vi "extract full and sub movement sequences.vi"(8 "end points in":i32[](array[numeric]), 9 "Start points in":i32[](array[numeric]), 11 "player movement data":i32[](array[numeric])) -> (2 "Sub patterns":string[](array[string]), 3 "Full movement patterns":string[](array[string]))   [LabVIEW 2013]
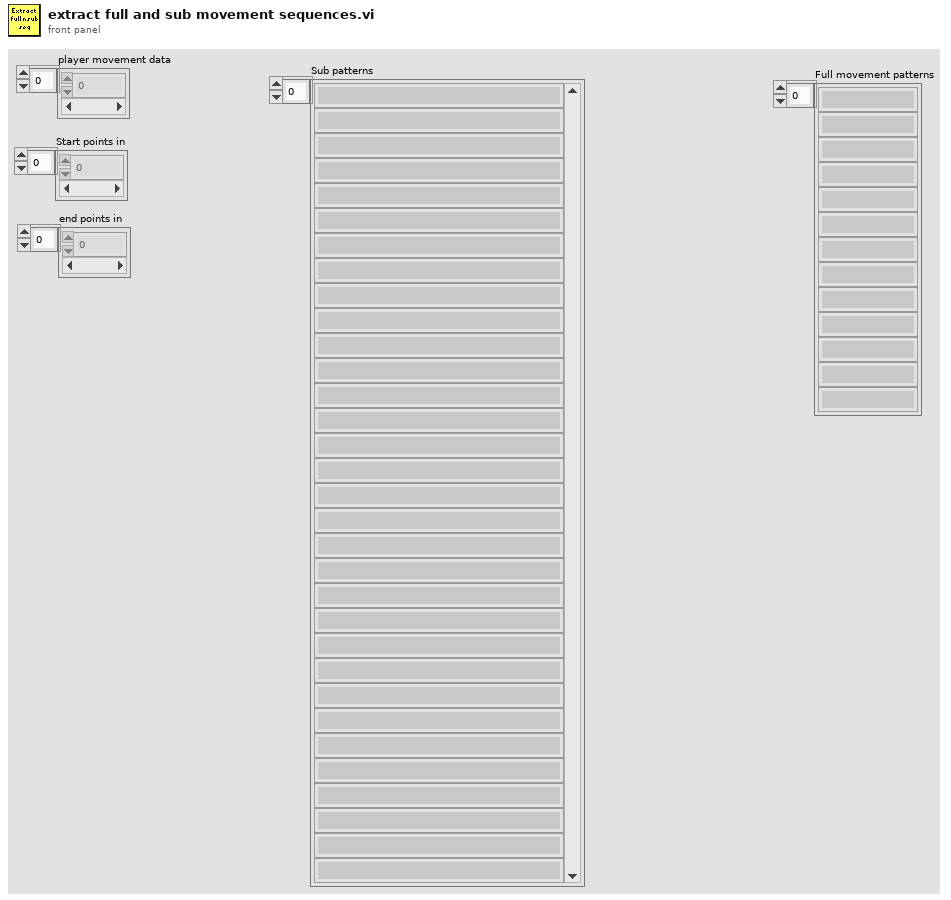
[diagram p1: front panel]
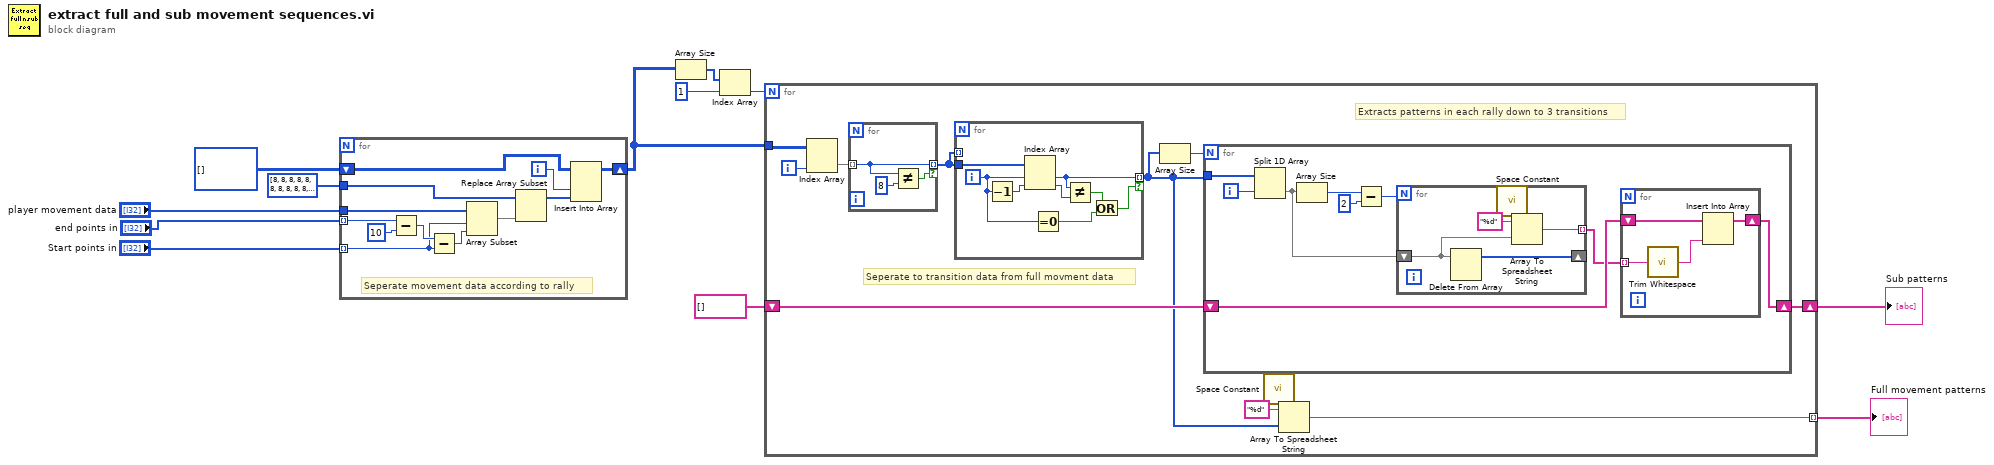
[diagram p0: block diagram]
diagram:
  n1 = for {
    tunnel: i32[] [8, 8, 8, 8, 8, 8, 8, 8, 8, 8, 8, 8, 8, 8, 8, 8, 8, 8, 8, 8, 8, 8, 8, 8, 8, 8, 8, 8, 8, 8, 8, 8, 8, 8, 8, 8, 8, 8, 8, 8, 8, 8, 8, 8, 8, 8, 8, 8, 8, 8, 8, 8, 8, 8, 8, 8, 8, 8, 8, 8, 8, 8, 8, 8, 8, 8, 8, 8, 8, 8, 8, 8, 8, 8, 8, 8, 8, 8, 8, 8, 8, 8, 8, 8, 8, 8, 8, 8, 8, 8, 8, 8, 8, 8, 8, 8, 8, 8, 8, 8, 8, 8, 8, 8, 8, 8, 8, 8, 8, 8, 8, 8, 8, 8, 8, 8, 8, 8, 8, 8, 8, 8, 8, 8, 8, 8, 8, 8, 8, 8, 8, 8, 8, 8, 8, 8, 8, 8, 8, 8, 8, 8, 8, 8, 8, 8, 8, 8, 8, 8, 8, 8, 8, 8, 8, 8, 8, 8, 8, 8, 8, 8, 8, 8, 8, 8, 8, 8, 8, 8, 8, 8, 8, 8, 8, 8, 8, 8, 8, 8, 8, 8, 8, 8, 8, 8, 8, 8, 8, 8, 8, 8, 8, 8, 8, 8, 8, 8, 8, 8, 8, 8, 8, 8, 8, 8, 8, 8, 8, 8, 8, 8, 8, 8, 8, 8, 8, 8, 8, 8, 8, 8, 8, 8, 8, 8, 8, 8, 8, 8, 8, 8, 8, 8, 8, 8, 8, 8, 8, 8, 8, 8, 8, 8, 8, 8, 8, 8, 8, 8, 8, 8, 8, 8, 8, 8, 8, 8, 8, 8, 8, 8, 8, 8, 8, 8, 8, 8, 8, 8, 8, 8, 8, 8, 8, 8, 8, 8, 8, 8, 8, 8, 8, 8, 8, 8, 8, 8, 8, 8, 8, 8, 8, 8, 8, 8, 8, 8, 8, 8, 8, 8, 8, 8, 8, 8, 8, 8, 8, 8, 8, 8, 8, 8, 8, 8, 8, 8, 8, 8, 8, 8, 8, 8, 8, 8, 8, 8, 8, 8, 8, 8, 8, 8, 8, 8, 8, 8, 8, 8, 8, 8, 8, 8, 8, 8, 8, 8, 8, 8, 8, 8, 8, 8, 8, 8, 8, 8, 8, 8, 8, 8, 8, 8, 8, 8, 8, 8, 8, 8, 8, 8, 8, 8, 8, 8, 8, 8, 8, 8, 8, 8, 8, 8, 8, 8, 8, 8, 8, 8, 8, 8, 8, 8, 8, 8, 8, 8, 8, 8, 8, 8, 8, 8, 8, 8, 8, 8, 8, 8, 8, 8, 8, 8, 8, 8, 8, 8, 8, 8, 8, 8, 8, 8, 8, 8, 8, 8, 8, 8, 8, 8, 8, 8, 8, 8, 8, 8, 8, 8, 8, 8, 8, 8, 8, 8, 8, 8, 8, 8, 8, 8, 8, 8, 8, 8, 8, 8, 8, 8, 8, 8, 8, 8, 8, 8, 8, 8, 8, 8, 8, 8, 8, 8, 8, 8, 8, 8, 8, 8, 8, 8, 8, 8, 8, 8, 8, 8, 8, 8, 8, 8, 8, 8, 8, 8, 8, 8, 8, 8, 8] -> [w20]
    tunnel: "end points in" -> [w24] mode=indexing
    tunnel: "Start points in" -> [w13] mode=indexing
    tunnel: "player movement data" -> [w22]
    shift-right: [w18] -> w3
    shift-left: i32[][] [] -> [w19]
    i -> [w15]
    # "Seperate movement data according to rally"
    n2 = Subtract(x=w24, y=10) -> (x-y=w14:i32)
    n3 = Subtract(x=w14, y=w13) -> (x-y=w21:i32)
    n4 = Array Subset(array=w22, index=w13, length=w21) -> (w16:i32[])
    n5 = Replace Array Subset(array=w20, new element=w16) -> (w17:i32[])  [unwired: 1 in]
    n6 = Insert Into Array(array=w19, index (col)=w15, new element=w17) -> (w18:i32[][])  [unwired: 1 in]
  }
  n7 = Array Size(array=w3) -> (size(s)=w9:i32[])
  n8 = Index Array(array=w9, index=1) -> (element=w4:i32)
  n9 = for {
    N: w4 -> [_]
    tunnel: w3 -> [w32]
    shift-right: [w35] -> w1
    shift-left: string[] [] -> [w31]
    tunnel: [w25] -> w2 mode=indexing
    i -> [w30]
    # "Extracts patterns in each rally down to 3 transitions"
    # "Seperate to transition data from full movment data"
    n10 = Index Array(array=w32, index (col)=w30) -> (element=w34:i32[])  [unwired: 1 in]
    n11 = for {
      tunnel: w34 -> [w46] mode=indexing
      tunnel: [w46] -> w33 mode=indexing if=w44
      n12 = Not Equal?(x=w46, y=8) -> (x != y?=w44:bool)
    }
    n13 = for {
      tunnel: w33 -> [_] mode=indexing
      tunnel: w33 -> [w43]
      tunnel: [w40] -> w26 mode=indexing if=w36
      i -> [w39]
      n14 = Decrement(x=w39) -> (x-1=w42:i32)
      n15 = Index Array(array=w43, index #1=w39, index #2=w42) -> (element #1=w40:i32, element #2=w41:i32)
      n16 = Equal To 0?(x=w39) -> (x = 0?=w37:bool)
      n17 = Not Equal?(x=w40, y=w41) -> (x != y?=w38:bool)
      n18 = Or(x=w38, y=w37) -> (x .or. y?=w36:bool)
    }
    n19 = Array Size(array=w26) -> (size(s)=w29:i32)
    n20 = for {
      N: w29 -> [_]
      tunnel: w26 -> [w50]
      shift-right: [w52] -> w35
      shift-left: w31 -> [w51]
      i -> [w49]
      n21 = Split 1D Array(array=w50, index=w49) -> (second subarray=w47:i32[])  [unwired: 1 out]
      n22 = Array Size(array=w47) -> (size(s)=w55:i32)
      n23 = Subtract(x=w55, y=2) -> (x-y=w53:i32)
      n24 = for {
        N: w53 -> [_]
        shift-right: [w61] -> _
        shift-left: w47 -> [w60]
        tunnel: [w62] -> w48 mode=indexing
        n25 = Delete From Array(array=w60) -> (array with subset deleted=w61:i32[])  [unwired: 2 in, 1 out]
        n26 = call <vilib>:"Space Constant.vi"() -> ("String"=w64:string)
        n27 = Array To Spreadsheet String(delimiter (Tab)=w64, array=w60, 3:"%d" ("format string")) -> (spreadsheet string=w62:string)
      }
      n28 = for {
        tunnel: w48 -> [w59] mode=indexing
        shift-right: [w56] -> w52
        shift-left: w51 -> [w58]
        n29 = call <vilib>:"Trim Whitespace.vi"("string"=w59) -> ("trimmed string"=w57:string)  [unwired: 1 in]
        n30 = Insert Into Array(array=w58, new element=w57) -> (w56:string[])  [unwired: 1 in]
      }
    }
    n31 = call <vilib>:"Space Constant.vi"() -> ("String"=w27:string)
    n32 = Array To Spreadsheet String(delimiter (Tab)=w27, array=w26, 3:"%d" ("format string")) -> (spreadsheet string=w25:string)
  }
  "Sub patterns" <- w1
  "Full movement patterns" <- w2
